vi "MAV_CMD_NAV_TAKEOFF.vi"(0 "Minimum Pitch":sgl, 1 "Aircraft ID":u8=1, 5 "Yaw Angle":sgl=284.0, 7 "Latitude":sgl, 9 "Longitude":sgl, 11 "Altitude (m)":sgl) -> (4 "MAVLink Message":u8[](array[numeric]))   [LabVIEW 2014]
panel:
  out "Payload Size":i32
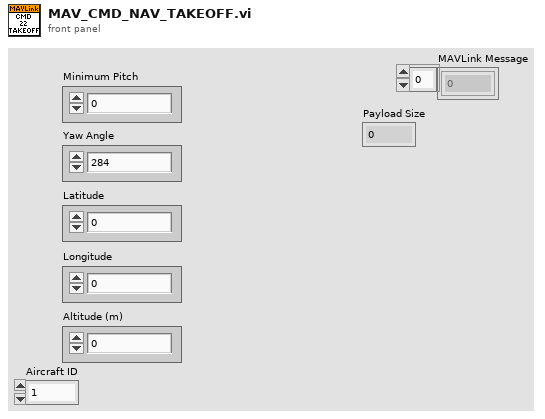
[diagram p1: front panel]
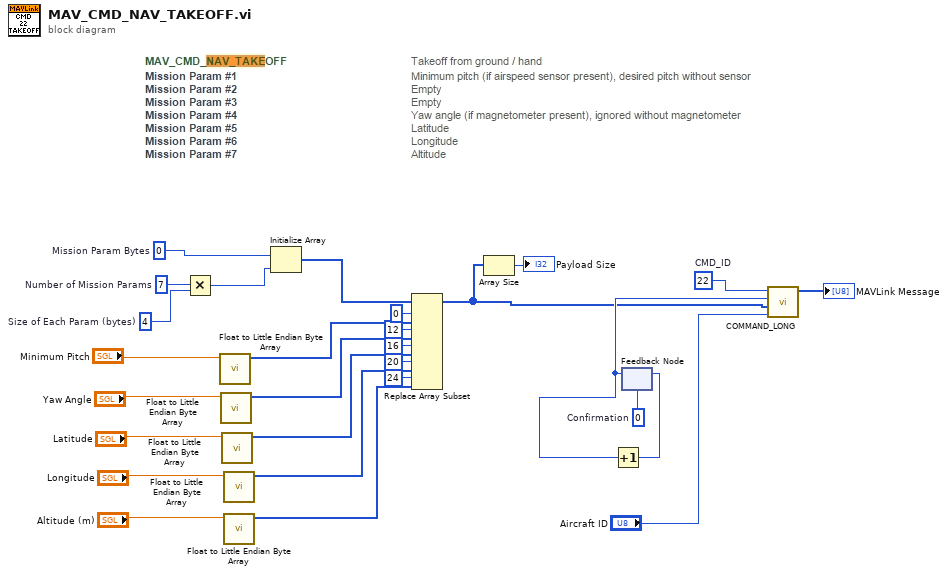
[diagram p0: block diagram]
diagram:
  w19 = u8 0  # Confirmation
  w26 = 4  # Size of Each Param (bytes)
  w27 = 7  # Number of Mission Params
  w28 = u8 0  # Mission Param Bytes
  w17 = u16 22  # CMD_ID
  n1 = Multiply(x=w27, y=w26) -> (x*y=w25:i32)
  n2 = call "Float to Little Endian Byte Array.vi"("Float In"="Minimum Pitch") -> ("LE Byte Array"=w11:u8[])  [unwired: 10 in]
  n3 = call "Float to Little Endian Byte Array.vi"("Float In"="Yaw Angle") -> ("LE Byte Array"=w10:u8[])  [unwired: 10 in]
  n4 = call "Float to Little Endian Byte Array.vi"("Float In"="Latitude") -> ("LE Byte Array"=w6:u8[])  [unwired: 10 in]
  n5 = call "Float to Little Endian Byte Array.vi"("Float In"="Longitude") -> ("LE Byte Array"=w4:u8[])  [unwired: 10 in]
  n6 = call "Float to Little Endian Byte Array.vi"("Float In"="Altitude (m)") -> ("LE Byte Array"=w2:u8[])  [unwired: 10 in]
  n7 = Initialize Array(w28, w25) -> (w24:u8[])
  n8 = Replace Array Subset(array=w24, new element #1=w11, index #1=0 ("index"), new element #2=w10, index #2=12 ("index"), new element #3=w6, index #3=16 ("index"), new element #4=w4, index #4=20 ("index"), new element #5=w2, index #5=24 ("index")) -> (w15:u8[])
  n9 = Array Size(array=w15) -> (size(s)=→"Payload Size":i32)
  n10 = feedback #1(w19) -> (w16:u8)
  n11 = Increment(x=w16) -> (x+1=w18:u8)
  n12 = feedback-in #1(w18) -> ()
  n13 = call "COMMAND_LONG.vi"("Target System and Target Component"="Aircraft ID", "Mission Params"=w15, "Confirmation"=w16, "Command ID"=w17) -> ("MAVLink Message"=→"MAVLink Message":u8[])  [unwired: 7 in]
